vi "_NiFpga_HdlFifo_GetBaseAddr.vi"(11 "Fifo Number":u32) -> (3 "Fifo Base Address":u32)   [LabVIEW 2023]
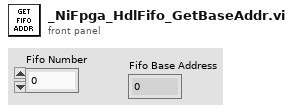
[diagram p1: front panel]
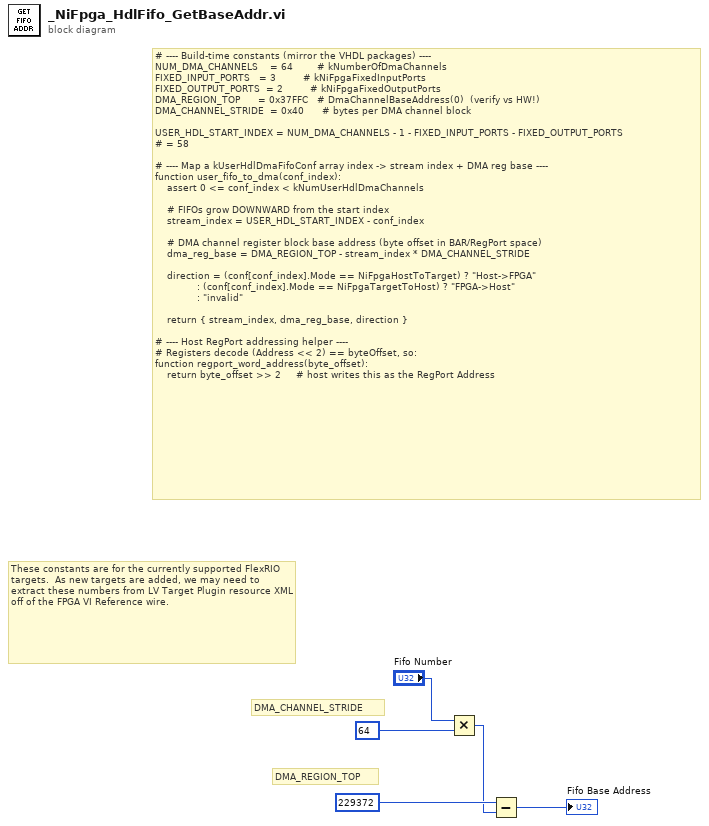
[diagram p0: block diagram]
diagram:
  # "DMA_CHANNEL_STRIDE"
  # "DMA_REGION_TOP"
  # "These constants are for the currently supported FlexRIO targets.  As new targets are added, we may need to extract these numbers from LV Target Plugin resource XML off of the FPGA VI Reference wire."
  # "# ---- Build-time constants (mirror the VHDL packages) ----\nNUM_DMA_CHANNELS    = 64        # kNumberOfDmaChannels\nFIXED_INPUT_PORTS   = 3         # kNiFpgaFixedInputPorts\nFIXED_OUTPUT_PORTS  = 2         # kNiFpgaFixedOutputPorts\nDMA_REGION_TOP      = 0x37FFC   # DmaChannelBaseAddress(0)  (verify vs HW!)\nDMA_CHANNEL_STRIDE  = 0x40      # bytes per DMA channel block\n\nUSER_HDL_START_INDEX = NUM_DMA_CHANNELS - 1 - FIXED_INPUT_PORTS - FIXED_OUTPUT_PORTS\n# = 58\n\n# ---- Map a kUserHdlDmaFifoConf array index -> stream index + DMA reg base ----\nfunction user_fifo_to_dma(conf_index):\n    assert 0 <= conf_index < kNumUserHdlDmaChannels\n\n    # FIFOs grow DOWNWARD from the start index\n    stream_index = USER_HDL_START_INDEX - conf_index\n\n    # DMA channel register block base address (byte offset in BAR/RegPort space)\n    dma_reg_base = DMA_REGION_TOP - stream_index * DMA_CHANNEL_STRIDE\n\n    direction = (conf[conf_index].Mode == NiFpgaHostToTarget) ? \"Host->FPGA\"\n              : (conf[conf_index].Mode == NiFpgaTargetToHost) ? \"FPGA->Host\"\n              : \"invalid\"\n\n    return { stream_index, dma_reg_base, direction }\n\n# ---- Host RegPort addressing helper ----\n# Registers decode (Address << 2) == byteOffset, so:\nfunction regport_word_address(byte_offset):\n    return byte_offset >> 2     # host writes this as the RegPort Address"
  n1 = Multiply(x="Fifo Number", y=u32 64 ("baseAddress")) -> (x*y=w3:u32)
  n2 = Subtract(x=u32 229372 ("baseAddress"), y=w3) -> (x-y=→"Fifo Base Address":u32)
